vi "超标留样通讯.vi"(8 "error in (no error)":errorcluster, 9 "VISA resource name":refnum<visa-resource-name> caption="VISA资源名称", 10 "写入缓冲区":string, 11 "功能输入":enum16{"打开串口", "写入", "读取", "关闭串口"}(ring)) -> (0 "error out":errorcluster, 2 "读取缓冲区":string, 3 "VISA resource name out":refnum<visa-resource-name>)   [LabVIEW 2016, in "科盛超标留样.lvlib"]
uses:
  <vilib>/Instr/_visa.llb/VISA Configure Serial Port (Instr).vi
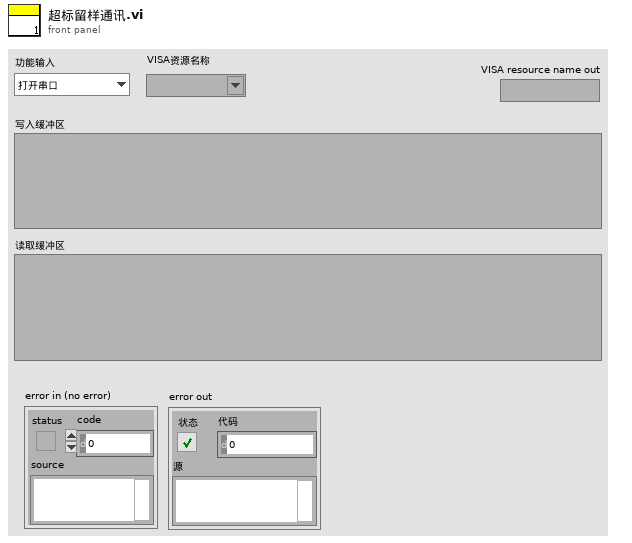
[diagram p1: front panel]
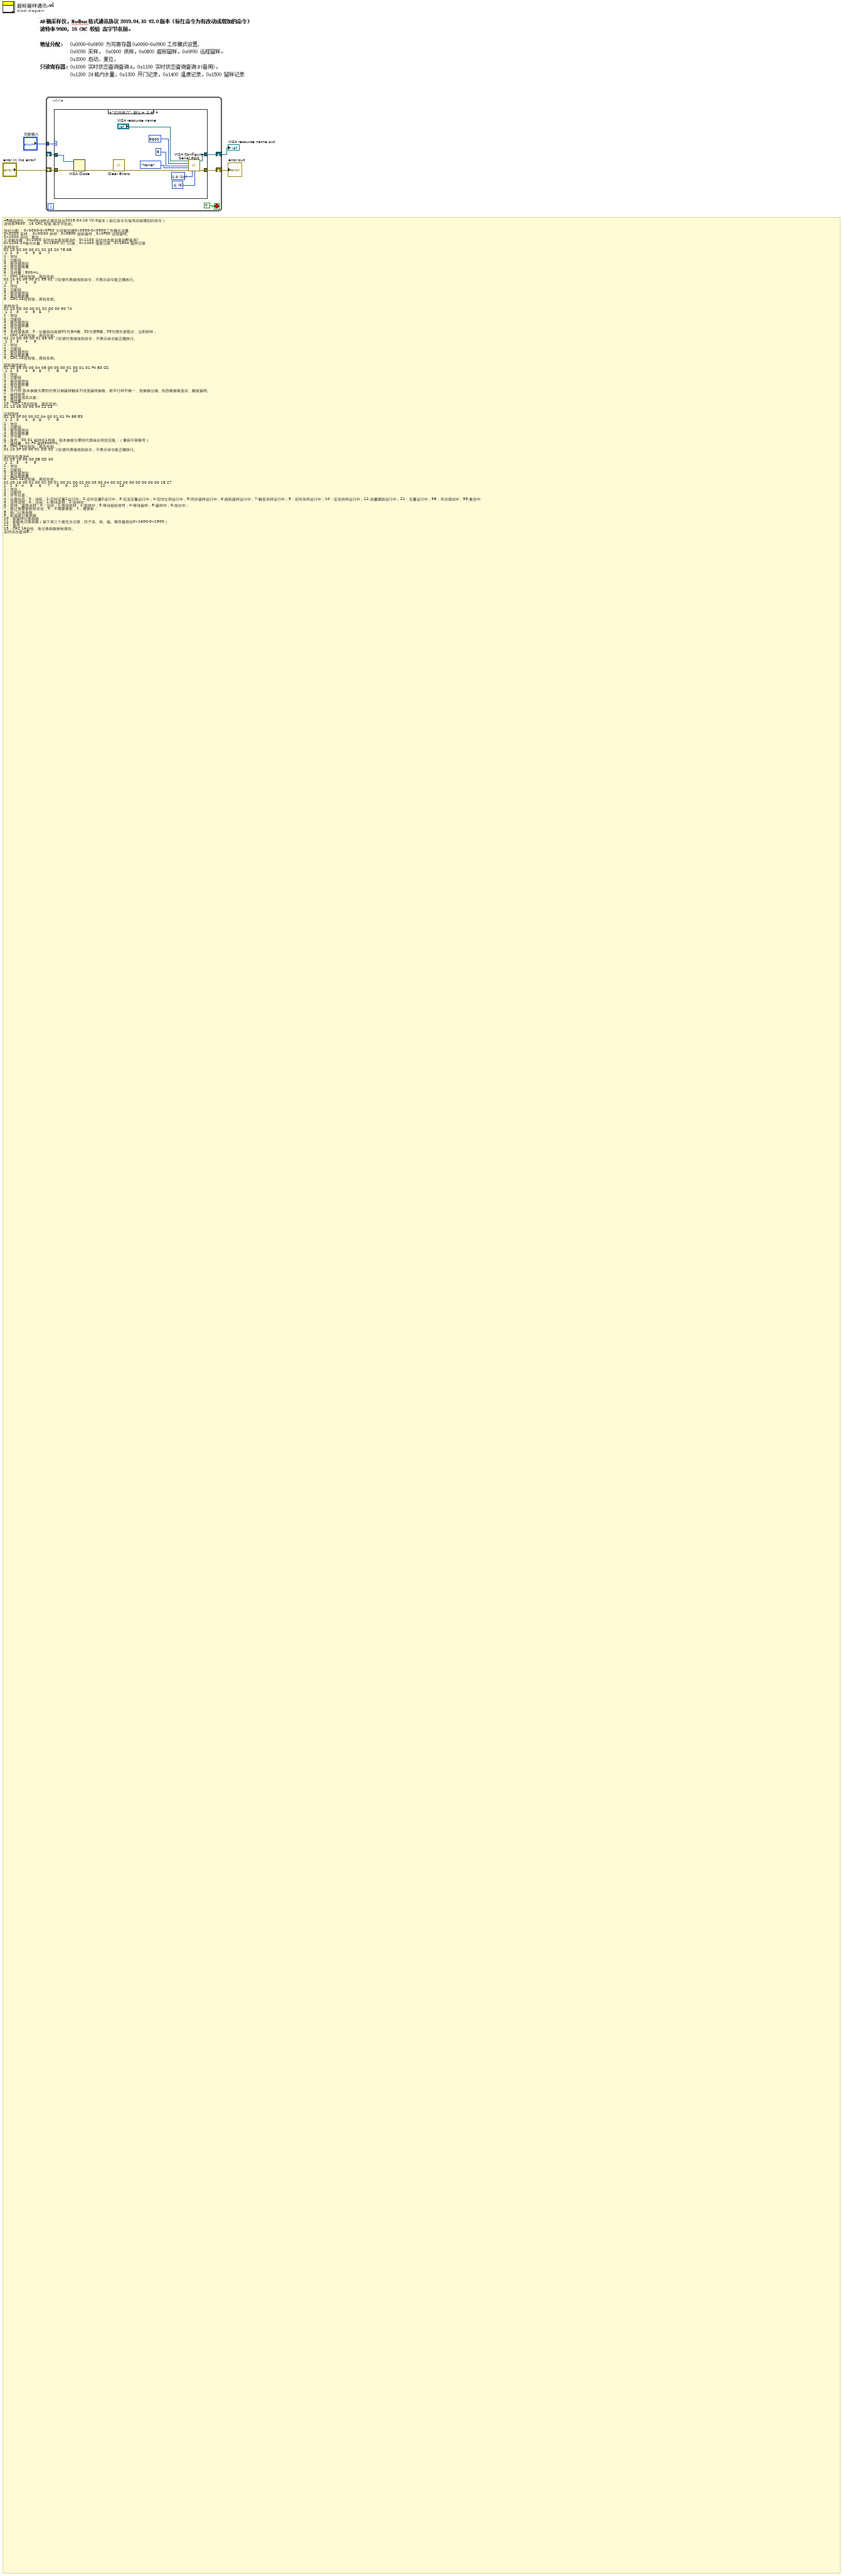
[diagram p0: block diagram]
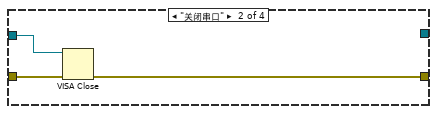
[diagram p2: hidden frame]
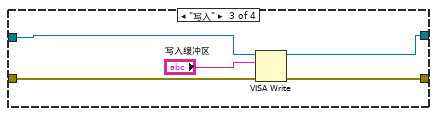
[diagram p3: hidden frame]
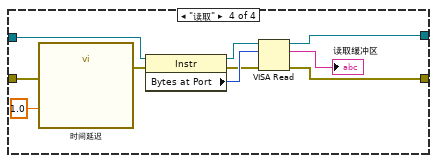
[diagram p4: hidden frame]
diagram:
  # "AB桶采样仪，Modbus格式通讯协议2019.04.10 V2.0版本（标红命令为有改动或增加的命令）\n波特率9600，16 CRC 校验 高字节在前。\n\n地址分配：\t0x0000-0x0F00 为写寄存器0x0000-0x0900工作模式设置, \n0x0C00 采样， 0x0D00 供样，0x0E00 超标留样，0x0F00 远程留样。\n0x2000 启动、复位，\n只读寄存器：0x1000 实时状态查询查询A，0x1100 实时状态查询查询B(备用)，\n0x1200 24瓶内水量，0x1300 开门记录，0x1400 温度记录，0x1500 留样记录\n采样命令\n01 10 0C 00 00 01 02 03 20 78 6B \n 1  2   3     4    5   6     7\n1：地址\n2：功能码 \n3：寄存器地址\n4：寄存器数量\n5：字节数；\n6：采样量；800mL；\n7：CRC 16位校验，高位在前。\n01 10 0C 00 00 01 99 02  //反馈代表接收到命令，不表示命令能正确执行。\n 1  2   3     4     5\n1：地址\n2：功能码\n3：寄存器地址  \n4：寄存器数量\n5：CRC 16位校验，高位在前。\n\n供样命令\n01 10 0D 00 00 01 02 00 00 90 7A \n 1  2   3     4    5   6     7\n1：地址\n2：功能码 \n3：寄存器地址\n4：寄存器数量\n5：字节数；\n6：供样源选择；0：仪器自动选择01代表A桶，02代表B桶，03代表外部取水，立即供样；\n7：CRC 16位校验，高位在前。\n01 10 0D 00 00 01 65 03  //反馈代表接收到命令，不表示命令能正确执行。\n 1  2   3     4     5\n1：地址\n2：功能码\n3：寄存器地址  \n4：寄存器数量\n5：CRC 16位校验，高位在前。\n\n超标留样命令\n01 10 0E 00 00 04 08 00 00 00 01 00 01 01 F4 E3 CC \n 1  2   3     4    5   6     7     8     9    10\n1：地址\n2：功能码\n3：寄存器地址 \n4：寄存器数量\n5：字节数；\n6：平行样,若本参数为零则代表只做留样触发不改变留样参数；若平行样不唯一，但参数出错，则忽略参数变动，触发留样。\n7：留样瓶号；\n8：留样瓶混采次数；\n9：留样量；\n10：CRC 16位校验，高位在前。\n01 10 0E 00 00 04 22 C3\n\n远程取样\n01 10 0F 00 00 02 04 00 01 01 F4 88 E3 \n 1  2   3     4    5   6     7     8\n1：地址\n2：功能码 \n3：寄存器地址\n4：寄存器数量\n5：字节数；   \n6：瓶号；00 01 留样在1号瓶；若本参数为零则代表自动寻找空瓶；（兼容不带瓶号）\n7：留样量；01 F4 留样500mL；\n8：CRC 16位校验，高位在前。\n01 10 0F 00 00 01 DD 02  //反馈代表接收到命令，不表示命令能正确执行。\n\n实时状态查询A\n01 03 10 00 00 0B CD 00  \n 1  2   3     4     5\n1：地址\n2：功能码\n3：寄存器地址\n4：寄存器数量\n5：CRC 16位校验，高位在前。\n01 03 16 00 01 00 01 00 01 00 01 00 02 00 03 00 04 00 02 00 00 00 00 00 00 18 27 \n1   2  3   4     5     6     7     8     9    10     11         12           13 \n1：地址；\n2：功能码；\n3：字节长度；\n4：仪器状态；0：待机；1:定时定量1运行中；2:定时定量2运行中；3:定流定量运行中；4:定时比例运行中；5:同步留样运行中；6:超标留样运行中；7:触发采样运行中；9：定时采样运行中；10：定流供样运行中；11:流量跟踪运行中；21：定量运行中；98：手动调试中；99:复位中\n5：采样流程；0：空闲；1:等待采样；2:采样中；\n6：供样、留样流程；0：空闲；1:等待供样；2:供样中；3:等待超标信号；4:等待留样；5:留样中；6:排水中；\n7：瓶记录需更新标志位，0：不需要更新，1：需更新；\n8：新门记录条数\n9：新温度记录条数\n10：新留样记录条数\n11：新断电记录条数（接下来三个是无水记录，对于采、供、留。寄存器地址0x1600-0x1900）\n12：备用；\n13：CRC 16位校\t\t\t各记录条数掉电保存。\n实时状态查询B\n01 03 11 00 00 11 FA 80  \n 1  2   3     4     5\n1：地址\n2：功能码\n3：寄存器地址\n4：寄存器数量\n5：CRC 16位校验，高位在前。\n01 03 22 0012 0006 0006 000A 000C 0000 0BB8 1388 002D 0032 0064 000A FFFF FFFF 0000 0000 0000 XX XX \n1  2  3               4                 5    6    7    8    9   10     11           12        13 \n1：地址；\n2：功能码；\n3：字节长度；\n4：仪器时间：18年6月6号10时12分00秒；\n5：采样桶水量：3000ml；\n6：供样桶水量：5000ml；\n7：冷藏箱温度：4.5℃，带一位小数；\n8：瞬时流速：50m3/h；\n9：COD值：100mg/L；\n10 NH3值：10mg/L；\n11：仪器部件状态：为二进制位共四个字节3-0；\n最高字节，第三字节。\n位\n电平\t7\t6\t5\t4\t3\t2\t1\t0\n1（高电）\t未定义\t未定义\t未定义\t未定义\t未定义\t未定义\t未定义\tA供B采\n0（低电）\t未定义\t未定义\t未定义\t未定义\t未定义\t未定义\t未定义\tA采B供\n第二字节，表示开关量状态：\n位\n电平\t7\t6\t5\t4\t3\t2\t1\t0\n1（高电）\t干簧管断开\t门关\tA浮球断开\tB浮球断开\t同步开关量断开\t超标开关量断开\t夹管阀1关\t夹管阀2关\n0（低电）\t干簧管闭合\t门开\tA浮球闭合/水满\tB浮球闭合/水满\t同步开关量闭合\t超标开关量闭合\t夹管阀1开\t夹管阀2开\n第一字节，表示器件运行状态：\n位\n电平\t7\t6\t5\t4\t3\t2\t1\t0\n1（高电）\t采样泵停\t供样泵停\t泵反转\tA桶搅拌关\tB桶搅拌关\t电控锁关\t准备好断开\t外控泵关\n0（低电）\t采样泵转\t供样泵转\t泵正转\tA桶搅拌开\tB桶搅拌关\t电控锁开\t准备好闭合\t外控泵开\n第零字节，表示阀状态：\n位\n电平\t7\t6\t5\t4\t3\t2\t1\t0\n1（高电）\tA桶阀关\tB桶阀关\t备用阀关\t冲洗阀关\t排水阀关\t供样阀关\t采样阀关\t进水阀关\n0（低电）\tA桶阀开\tB桶阀开\t未用，常为1\t未用，常为1\t排水阀开\t供样阀开\t采样阀开\t进水阀开\n12：备用；\n13：CRC 16位校\n\n查询24留样瓶水量\n 01 03 12 00 00 18 B8 40  \n  1  2   3     4     5\n4：寄存器数量，共24个留样瓶，每瓶水量占一个寄存器长度。\n 01 03 30 01 F4 00 64 00 00  ...  XX XX  \n  1  2  3   4     5     6          28  \n1：地址；\n2：功能码；\n3：字节长度；\n4-27：对应1-24号留样瓶内水量；\n28：CRC 16位校验\n\n开门记录查询\n01 03 13 00 00 07 XX XX //01 03 13 00 00 0E  8A C0   查询两条记录\n 1  2   3     4     5\n4：寄存器数量，通过实时状态查询A命令获得记录条数，每条记录占7个寄存器长度。\n01 03 0E 0012 0006 0006 000A 000C 0000 0001 XX XX \n 1  2  3               4                5     6  \n1：地址；\n2：功能码；\n3：字节长度；\n4：开门时间；0012 0006 0006 000A 000C 0000 ，18年6月6号10时12分0秒\n5：开门状态；1开门，0关门\n6：CRC 16位校验\n\n温度记录查询\n01 03 14 00 00 07 XX XX\n 1  2   3     4     5\n4：寄存器数量，通过实时状态查询A命令获得记录条数，每条记录占7个寄存器长度。\n01 03 0E 0012 0006 0006 000A 000C 0000 0001 XX XX  \n 1  2  3               4                5     6  \n1：地址；\n2：功能码；\n3：字节长度；\n4：记录时间；0012 0006 0006 000A 000C 0000 ，18年6月6号10时12分0秒\n5：冷藏状态；0超标，1冷藏\n6：CRC 16位校验\n\n留样记录查询\n01 03 15 00 00 0F XX XX \n 1  2   3     4     5\n4：寄存器数量，通过实时状态查询A命令获得记录条数，每条记录占15个寄存器长度。\n01 03 1E 0012 0006 0006 000A 000C 0000 00 01 00 01 00 01 00 02 00 01 00 02\n 1  2  3               4                 5     6        7           8      \n00 01 00 64 00 C8 XX XX     \n    9    10    11    12\n1：地址；\n2：功能码；\n3：字节长度；\n4：采样发生时间，即15年6月6日10时11分00秒；（兼容原协议，默认秒一直为0）\n5：采样模式：0:定时定量1；1:定时定量2；2:定流定量；3:定时比例；4:同步留样；5:超标留样；6:触发采样；7:定时采样1；8：定时采样2；9：定流供样；10:流量跟踪；20：定量；97:mA触发留样98:远程取样99:手动调试\n6：此次采样在1号瓶进行；\n7：当前混采1次，设定混采2次；\n8：当前瓶号平行样为1，设定平行样为2。\n9：超标信息，当前瓶超标留样信号：1开关量，2 COD模拟量,3氨氮模拟量，4串口。\n10：当次采样量为100ml；\n11：当前瓶内总水样量为200ml；\n12：CRC 16位校验\n\n关于查询命令：\n24瓶留样瓶记录是长度固定的，每次返回24瓶记录。开门记录和温度记录长度14个字节，每多查到一条记录即增加14个字节，记录不超过十条以控制长度在145字节以内。留样记录长度30字节，每多查到一条记录即增加30个字节长度，记录不超过5条，以控制长度不超过155字节。\n三个长度可变的记录的新增记录条数在实时状态查询中有体现.\n\n\n定点定量\n01 10 00 00 00 36 6C 00 02 00 01 00 18 00 02 01 2C 00 7F 00 00 00 0F 00 00 00 2D 00 01 00 0F\n1  2   3     4    5   6     7     8     9    10    11      12                     \n00 01 00 2D 00 02 00 0F 00 02 00 2D 00 03 00 0F 00 03 00 2D 00 04 00 0F 00 04 00 2D 00 05 00 0F \n00 05 00 2D 00 06 00 0F 00 06 00 2D 00 07 00 0F 00 07 00 2D 00 08 00 0F 00 08 00 2D 00 09 00 0F \n00 09 00 2D 00 0A 00 0F 00 0A 00 2D 00 0B 00 0F 00 0B 00 2D XX XX \n1：地址\n2：功能码 \n3：寄存器地址\n4：寄存器数量\n5：字节数；\n6：02 表示一次取水样中会依次给两个瓶内采水；\n7：01表示留样从1号瓶开始；\n8：18表示留样在24号瓶结束；\n9：02表示每个采样瓶中混采2次；\n10：01 2C 表示定时时刻到后留样瓶留样300ml；\n11：以二进制的方式控制一周七天的循环采样开启情况，0x7F = 0111 1111代表七天都开启留样；\n12：00 00 00 0F ...表示定时的时间为00时15分，定时时刻一共24组。00时00分为无效时间。\n13：XX XX ,CRC 16位校验，高位在前。\n01 10 00 00 00 36 1F 40  //反馈代表接收到命令，不表示命令能正确执行。\n\n定时定量\n01 10 01 00 00 06 0C 00 02 00 01 00 18 00 02 01 2C 00 3C XX XX\n1  2   3     4    5    6    7     8     9     10    11    12             \n1：地址\n2：功能码 \n3：寄存器地址\n4：寄存器数量\n5：字节数；\n6：02 表示一次取水样中会依次给两个瓶内采水；\n7：01表示留样从1号瓶开始；\n8：18表示留样在24号瓶结束；\n9：02表示每个采样瓶中混采2次；\n10：01 2C 表示定时间隔到后留样瓶留样300ml；\n11：00 3C 表示每隔60分钟留样一次。\n13：XX XX ,CRC 16位校验，高位在前。\n01 10 01 00 00 06 F7 41  //反馈代表接收到命令，不表示命令能正确执行。\n\n定流定量\n01 10 02 00 00 07 0E 00 02 00 01 00 18 00 02 01 2C 00 00 00 64 XX XX\n1  2   3     4    5    6    7     8     9     10       11       12             \n1：地址\n2：功能码 \n3：寄存器地址\n4：寄存器数量\n5：字节数；\n6：02 表示一次取水样中会依次给两个瓶内采水；\n7：01表示留样从1号瓶开始；\n8：18表示留样在24号瓶结束；\n9：02表示每个采样瓶中混采2次；\n10：01 2C 表示累计设定的流量后留样瓶留样300ml；\n11：00 00 00 64 表示每累计100m3，采样一次。此数据最大为5位十进制数：99999。\n12：XX XX ,CRC 16位校验，高位在前。\n01 10 02 00 00 07 73 80  //反馈代表接收到命令，不表示命令能正确执行。\n\n定时比例\n01 10 03 00 00 07 0E 00 02 00 01 00 18 00 02 00 3C 00 01 86 A0 XX XX\n1  2   3     4    5    6    7     8     9     10       11       12             \n1：地址\n2：功能码 \n3：寄存器地址\n4：寄存器数量\n5：字节数；\n6：02 表示一次取水样中会依次给两个瓶内采水；\n7：01表示留样从1号瓶开始；\n8：18表示留样在24号瓶结束；\n9：02表示每个采样瓶中混采2次；\n10：00 3C 表示累计流量60分钟，根据累计的流量和第11部分的比例计算采样量；\n11：00 01 86 A0 表示换算比例为1/100000，即每累计1m3，采样10ml水样。此数据最大为8位十进制数：9999 9999。\n12：XX XX ,CRC 16位校验，高位在前。\n01 10 03 00 00 07 8F 81  //反馈代表接收到命令，不表示命令能正确执行。\n\n同步留样\n01 10 04 00 00 05 0A 00 02 00 01 00 18 00 02 01 2C XX XX\n1  2   3     4    5    6    7     8     9     10    11               \n1：地址\n2：功能码 \n3：寄存器地址\n4：寄存器数量\n5：字节数；\n6：02 表示一次取水样中会依次给两个瓶内采水；\n7：01表示留样从1号瓶开始；\n8：18表示留样在24号瓶结束；\n9：02表示每个采样瓶中混采2次；\n10：01 2C 表示接收一次同步信号后留样瓶留样300ml；\n11：XX XX ,CRC 16位校验，高位在前。\n同步留样中，在等待同步信号时，收到本地留样命令亦可触发留样（只做触发）。\n01 10 04 00 00 05 3A 01  //反馈代表接收到命令，不表示命令能正确执行。\n\n\n超标留样\n01 10 05 00 00 0B 16 00 02 00 01 00 18 00 02 01 2C 00 3C 00 64 03 E8 01 F4 03 E8 01 F4 XX XX\n1  2   3     4    5   6     7   \t8      9    10    11    12     13   14    15    16    17\n1：地址\n2：功能码 \n3：寄存器地址\n4：寄存器数量\n5：字节数；\n6：02 表示一次取水样中会依次给两个瓶内采水；\n7：01表示留样从1号瓶开始；\n8：18表示留样在24号瓶结束；\n9：02表示每个采样瓶中混采2次；\n10：01 2C 表示收到超标信号后留样瓶留样300ml；\n11：00 3C 表示每隔60分钟，往留样桶中进水；\n12：00 14 表示等待超标信号20秒，超过时间则排空缓冲杯,此数据最大为2位十进制数：99；\n13：03 E8 表示COD模拟量信号输入，20mA模拟量对应值1000mg/L；\n14：01 F4表示输入的COD模拟信号，根据20mA值转换后，达到500mg/L则触发超标采样；\n15：03 E8 表示NH3模拟量信号输入，20mA模拟量对应值1000mg/L；\n16：01 F4表示输入的NH3模拟信号，根据20mA值转换后，达到500mg/L则触发超标采样；\n17：XX XX ,CRC 16位校验，高位在前。\n01 10 05 00 00 0B 02 81  //反馈代表接收到命令，不表示命令能正确执行。\n\n\n触发采样\n01 10 06 00 00 04 08 00 01 00 78 00 5A 00 1E XX XX\n1  2   3     4    5   6     7     8     9     10     \n1：地址\n2：功能码 \n3：寄存器地址\n4：寄存器数量\n5：字节数；\n6：01表示采样桶设定为A桶，若为02则为B桶；若此参数为零表示本命令只做启动触发采样（运行中）/触发采样（待机），不修改采样参数；\n7：00 78 表示在一次同步触发后隔120分钟，再次等待同步触发往混匀桶中进水；\n8：00 5A 表示供样后等待超标信号90分钟，超过此时间则排空缓冲杯，需小于采样间隔10分钟。此数据最大为3位十进制数：999；\n9：00 1E 表示留样桶满后和往采样瓶采水前都搅拌均质30秒，此数据最大为3位十进制数：999；\n10：XX XX ,CRC 16位校验，高位在前。\n01 10 06 00 00 04 42 C1  //反馈代表接收到命令，不表示命令能正确执行。\n\n\n定时采样\n01 10 08 00 00 06 0C 00 01 00 78 00 01 00 32 00 5A 00 1E XX XX\n1  2   3     4    5   6     7     8     9     10    11    12\n1：地址\n2：功能码 \n3：寄存器地址\n4：寄存器数量\n5：字节数；\n6：01表示留样桶设定为A桶，若为02则为B桶；若此参数为零表示本命令只做启动定时采样，不修改采样参数；\n7：00 78表示水质分析仪器预计的取样周期是120分钟，则本仪器的供样周期也是120分钟；\n8：01 表示为定采样间隔设置，02表示为定预采样量设置，在供样周期内，缓冲杯需预采样5L以确保供样时水样\t足够。定采样间隔，则根据供样周期及采样间隔，计算出采集5L水样，每次需采集多少水样；定预采样量，\t则根据供样周期及预采样量，计算出采集5L水样，每次采样间隔几分钟。\n9：00 32 \t1、若第四部分设置为定采样间隔，表示每隔50分钟，往留样桶中进水。\n   \t        2、若第四部分设置为定预采样量，表示每次往缓冲杯采集50mL水样（水量不可小于200ml，此处用\t同一参数，解释两种情况下参数的含义）；\n10：00 5A表示供样后等待超标信号90分钟，超过时间则排空缓冲杯，此数据最大为3位十进制数：999；\n11：00 1E 表示留样桶满后和往采样瓶采水前都搅拌均质30秒，此数据为3位，最高位无效。\n12：XX XX ,CRC 16位校验，高位在前。\n01 10 08 00 00 06 6B 42  //反馈代表接收到命令，不表示命令能正确执行。\n\n定流采样\n01 10 09 00 00 06 0C 00 02 00 00 00 0A 01 2C 00 5A 00 1E XX XX\n1  2   3     4    5   6        7        8      9    10    11   \n1：地址\n2：功能码 \n3：寄存器地址\n4：寄存器数量\n5：字节数；\n6：01表示留样桶设定为A桶，若为02则为B桶；若此参数为零表示本命令只做启动定流采样，不修改采样参数；\n7：00 00 00 0A 表示每累计10m3，往留样桶中进水，此数据最大为5位十进制数：99999；\n8：01 2C 表示每累计设定的流量值，往混匀桶中进水300ml\n9：00 5A 表示供样后等待超标信号90分钟，超过时间则排空缓冲杯，此数据最大为3位十进制数：999；\n10：00 1E 表示留样桶满后和往采样瓶采水前都搅拌均质30秒，此数据为3位，最高位无效。\n11：XX XX ,CRC 16位校验，高位在前。\n01 10 09 00 00 06 97 43  //反馈代表接收到命令，不表示命令能正确执行。\n\n启动、复位、开门\n01 10 20 00 00 01 02 00 01 52 46 （启动）//01 10 20 00 00 01 02 00 02 53 06 (复位)\n 1  2   3     4    5   6     7\n1：地址\n2：功能码 \n3：寄存器地址\n4：寄存器数量\n5：字节数；\n6：操作选择；01代表启动，02代表复位，10 代表开门；（门开状态下，未解锁键盘也可按键清空瓶记录）\n7：CRC 16位校验，高位在前。\n01 10 0C 00 00 01 99 02  //反馈代表接收到命令，不表示命令能正确执行。\n将Factory_set2 Bit0位置一，写寄存器操作反馈增加命令检查标志位。//01成功02系统忙（已运行）03参数检查错误04控制时序错误（采样、供样、留样）"
  n1 = while {
    shift-right: [w9] -> w1
    shift-left: _ -> [w7]
    shift-right: [w8] -> w2
    shift-left: "error in (no error)" -> [w6]
    tunnel: "功能输入" -> [w5]
    stop <- TRUE stop-if-true
    n2 = case shown="\"打开串口\", 默认" w5 {
      tunnel: [w13 _ w28 w39] -> w9
      tunnel: [w12 w25 w27 w38] -> w8
      tunnel: w7 -> [w21 w24 w30 w36]
      tunnel: w6 -> [w22 w23 w29 w40]
      frame "打开串口", Default {
        w14 = u16 0 items=["无", "XON/XOFF", "RTS/CTS", "XON/XOFF & RTS/CTS", "DTR/DSR", "XON/XOFF & DTR/DSR"] ("flow control (0:none)")
        w16 = u16 10 items=["1.0"=10, "1.5"=15, "2.0"=20] ("stop bits (10: 1 bit)")
        n3 = VISA Close(VISA resource name=w21, error in (no error)=w22) -> (error out=w20:errorcluster)
        n4 = call <vilib>:"Clear Errors.vi"("error in (no error)"=w20) -> ("error out"=w19:errorcluster)  [unwired: 5 in, 1 out]
        n5 = call-poly "VISA Configure Serial Port"("VISA resource name"="VISA resource name", "baud rate (9600)"=u32 9600, "data bits (8)"=u16 8, "parity (0:none)"=enum16{"None", "Odd", "Even", "Mark", "Space"}."None", "error in (no error)"=w19, "stop bits (10: 1 bit)"=w16, "flow control (0:none)"=w14) -> ("VISA resource name out"=w13:refnum<visa-resource-name>, "error out"=w12:errorcluster)  [unwired: 7 in]
      }
      frame "关闭串口" {
        n6 = VISA Close(VISA resource name=w24, error in (no error)=w23) -> (error out=w25:errorcluster)
      }
      frame "写入" {
        n7 = VISA Write(VISA resource name=w30, write buffer="写入缓冲区", error in (no error)=w29) -> (VISA resource name out=w28:refnum<visa-resource-name>, error out=w27:errorcluster)  [unwired: 1 out]
      }
      frame "读取" {
        n8 = call "时间延迟"("error in (no error)"=w40, "Delay Time (s)"=1.0) -> ("error out"=w34:errorcluster)  [unwired: 9 in]
        n9 = property class="Instr"(reference=w36, error in=w34) -> (reference out=w32:refnum<visa-resource-name>, error out=w33:errorcluster, "Bytes at Port"=w35:u32)
        n10 = VISA Read(VISA resource name=w32, byte count=w35, error in (no error)=w33) -> (VISA resource name out=w39:refnum<visa-resource-name>, read buffer=→"读取缓冲区":string, error out=w38:errorcluster)  [unwired: 1 out]
      }
    }
  }
  "error out" <- w2
  "VISA resource name out" <- w1
